vi "WrapPolarPlot.vi"(11 "thetaRin":cluster{"Angle":dbl[], "Radius":dbl[]}) -> (3 "thetaRout":cluster{"Angle":dbl[], "Radius":dbl[]})   [LabVIEW 2012]
panel:
  out "gap":dbl
  in  "maxWrap":dbl=30.0
  out "max angle":dbl
  out "min angle":dbl
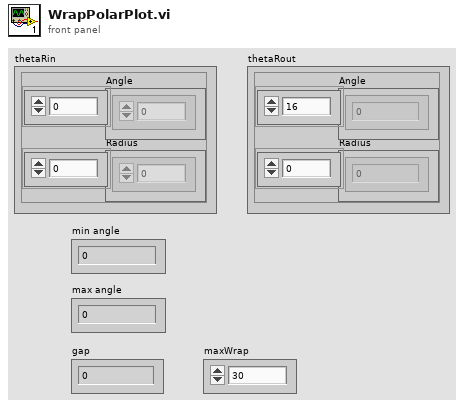
[diagram p1: front panel]
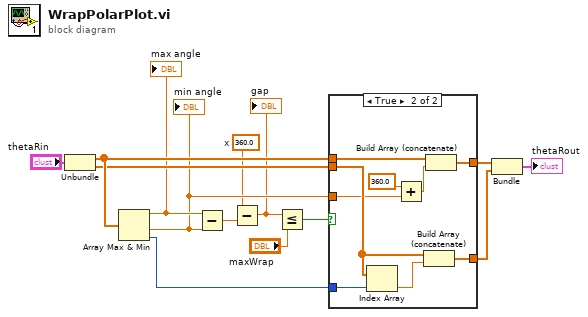
[diagram p0: block diagram]
diagram:
  w1 = 360.0  # x
  n1 = Unbundle("thetaRin") -> ("Angle"=w13:dbl[], "Radius"=w12:dbl[])
  n2 = Array Max & Min(array=w13) -> (max value=w7:dbl, min value=w4:dbl, min index (indices)=w14:i32)  [unwired: 1 out]
  "min angle" <- w4
  "max angle" <- w7
  n3 = Subtract(x=w7, y=w4) -> (x-y=w2:dbl)
  n4 = Subtract(x=w1, y=w2) -> (x-y=w3:dbl)
  "gap" <- w3
  n5 = Less Or Equal?(x=w3, y="maxWrap") -> (x <= y?=w5:bool)
  n6 = case shown="True" w5 {
    tunnel: [w15 w24] -> w10
    tunnel: w13 -> [w16 w23]
    tunnel: [w16 w22] -> w11
    tunnel: w12 -> [w15 w21]
    tunnel: w14 -> [_ w20]
    tunnel: w4 -> [_ w19]
    frame False {
    }
    frame True {
      n7 = Index Array(array=w21, index=w20) -> (element=w25:dbl)
      n8 = Add(x=360.0, y=w19) -> (x+y=w17:dbl)
      n9 = Build Array (concatenate)(w21, w25) -> (w24:dbl[])
      n10 = Build Array (concatenate)(w23, w17) -> (w22:dbl[])
    }
  }
  n11 = Bundle("Angle"=w11, "Radius"=w10) -> (→"thetaRout":cluster{"Angle":dbl[], "Radius":dbl[]})  [unwired: 1 in]
